vi "ROS_Topic_Write_Continuous_Primitive.vi"(2 "Msg in":string, 3 "ROS in":T1={"topic port"=0, "Node"="", "topic"="", "type"="", "node port"=0, "error "={"status"=FALSE, "code"=0, "source"=""}, "Direction"=enum."Node", "Update (ms)"=1, "FIFO size"=1}) -> (1 "ROS out":T1={"topic port"=0, "Node"="", "topic"="", "type"="", "node port"=0, "error "={"status"=FALSE, "code"=0, "source"=""}, "Direction"=enum."Node", "Update (ms)"=1, "FIFO size"=1})   [LabVIEW 2012]
doc: "Instructs the server to write out the data as often as possible. The server updates the message being sent upon a new ROS_Topic_Write call."
uses:
  <userlib>/ROS for LabVIEW Software/ROS/Code/SubVIs/_ROSControl.ctl
  <userlib>/ROS for LabVIEW Software/ROS/Code/SubVIs/_ROSDirection.ctl
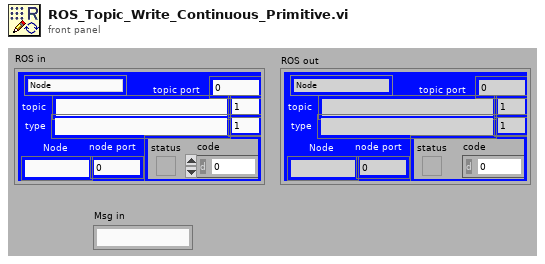
[diagram p1: front panel]
types:
  T1 = typedef "_ROSControl.ctl" = cluster{"topic port":u16, "Node":string, "topic":string, "type":string, "node port":u16, "error ":errorcluster, "Direction":T2, "Update (ms)":u16, "FIFO size":u16}
  T2 = typedef "_ROSDirection.ctl" = enum16{"Node", "Publisher", "Subscriber", "ServiceClient", "ServiceProvider"}
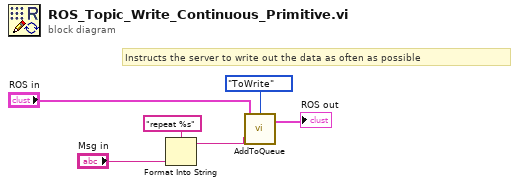
[diagram p0: block diagram]
diagram:
  # "Instructs the server to write out the data as often as possible"
  n1 = Format Into String(format string="repeat %s" ("name (unnamed)"), "Msg in") -> (resulting string=w4:string)  [unwired: 2 in, 1 out]
  n2 = call <userlib>:"AddToQueue.vi"("Cmd"=w4, "ROS"="ROS in", "Type"=enum16{"topic", "node", "ToFIFO", "ToWrite"}."ToWrite") -> ("ROS out"=→"ROS out":T1)  [unwired: 2 in]
